vi "test_Split Registers by Direction_Errors.vi"(8 "error in (no error)":errorcluster, 11 "TestCase in":refnum<class "FPGA Addon Load And Parse Bitfile Unit Tests.lvclass">) -> (0 "error out":errorcluster, 3 "TestCase out":refnum<class "FPGA Addon Load And Parse Bitfile Unit Tests.lvclass">)   [LabVIEW 2018, in "FPGA Addon Load And Parse Bitfile Unit Tests.lvclass"]
uses:
  FPGA Addon Load And Parse Bitfile Unit Tests.lvclass
  <vilib>/addons/_JKI Toolkits/VI Tester/TestCase.llb/TestCase.lvclass
  Addon/Addon System Explorer/FPGA Addon System Explorer.lvlib
  C:/Program Files (x86)/National Instruments/LabVIEW 2018/vi.lib/addons/_JKI Toolkits/VI Tester/TestCase.llb/TestCase.lvclass
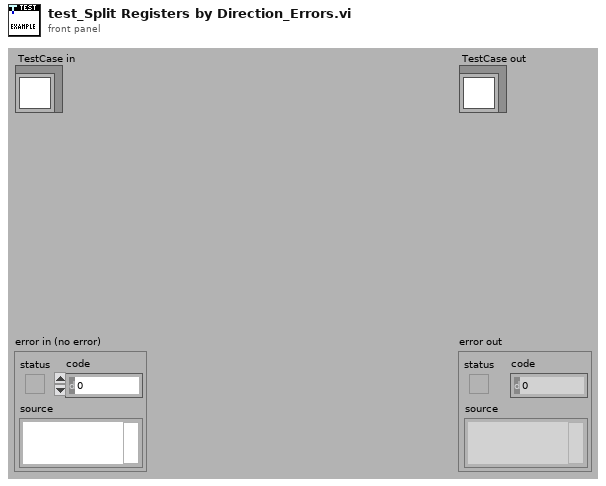
[diagram p1: front panel]
types:
  T1 = typedef "niFpgaBitfileStructure_VI.ctl" = cluster{"Name":string, "RegisterMap":T2[], "Icon":T7}
  T2 = typedef "nirviControlStructure.ctl" = cluster{"Name":string, "Hidden":bool, "Indicator":bool, "Flattened Type":string, "Grouping":cluster{"Grouped":bool, "Member Names":string[], "Member IDs":u32[]}, "Address":u32, "Size":u32, "Class":u32, "Internal":bool, "Typedef":T3, "ID":u32, "Bidirectional":bool, "Synchronous":bool, "Mechanical Action":T4, "Sub Controls":T5[], "Access May Timeout":bool, "Register Node":bool}
  T3 = typedef "nirviTypdefDescription.ctl" = cluster{"Typedef":bool, "Path":path}
  T4 = typedef "nirviMechanicalAction.ctl" = enum8{"Switch When Pressed", "Switch When Released", "Switch Until Released", "Latch When Pressed", "Latch When Released", "Latch Until Released"}
  T5 = typedef "nirviSubControlStructure.ctl" = cluster{"Name":string, "flattened Type":string, "Cluster Information":T6, "Typedef":T3}
  T6 = typedef "nirviClusterElementControl.ctl" = cluster{"Name Hierarchy":string[], "Item Order":u32[]}
  T7 = typedef "imagedata.ctl" = cluster{"image type":i32, "image depth":i32, "image":u8[], "mask":u8[], "colors":u32[], "Rectangle":cluster{"left":i16, "top":i16, "right":i16, "bottom":i16}}
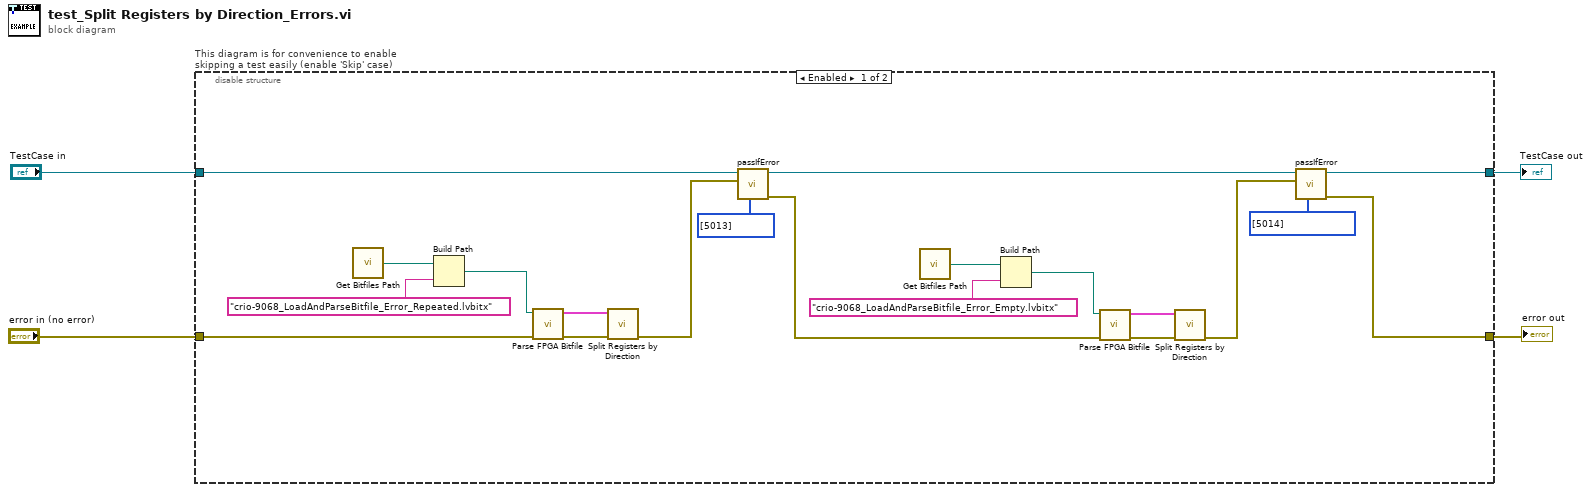
[diagram p0: block diagram]
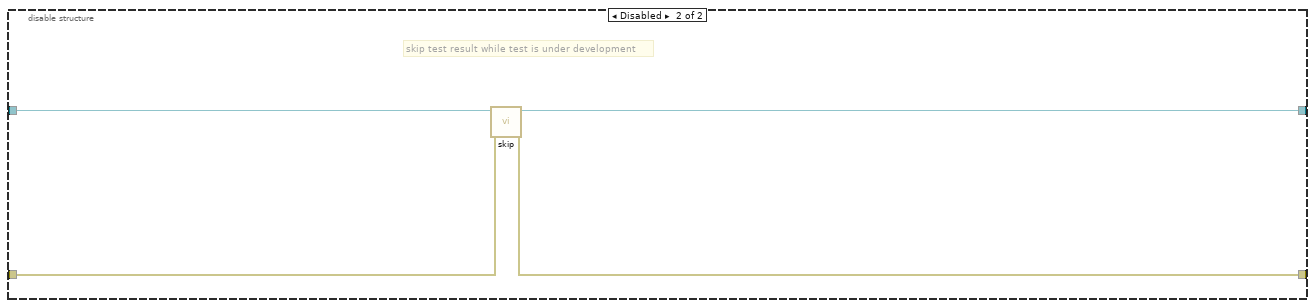
[diagram p2: hidden frame]
diagram:
  n1 = disable-structure "This diagram is for convenience to enable skipping a test easily (enable 'Skip' case)" shown="Enabled" {
    disable-tunnel: "TestCase in" -> [w18 w28]
    disable-tunnel: [w5 w26] -> w1
    disable-tunnel: [w6 w27] -> w3
    disable-tunnel: "error in (no error)" -> [w24 w25]
    frame Enabled {
      n2 = call "Get Bitfiles Path.vi"() -> ("Bitfiles path"=w21:path)
      n3 = Build Path(base path=w21, name or relative path="crio-9068_LoadAndParseBitfile_Error_Repeated.lvbitx") -> (appended path=w19:path)
      n4 = call "Parse FPGA Bitfile.vi"("error in (no error)"=w24, "Path"=w19) -> ("error out"=w23:errorcluster, "vi info"=w22:T1)  [unwired: 7 in, 1 out]
      n5 = call "Split Registers by Direction.vi"("error in"=w23, "vi info"=w22) -> ("error out"=w17:errorcluster)  [unwired: 7 in, 2 out]
      n6 = call-dynamic "passIfError.vi"("passing error codes (default = any error code)"=i32[] [5013], "error"=w17, "TestCase in"=w18) -> ("error out"=w10:errorcluster, "TestCase out"=w9:refnum<class "FPGA Addon Load And Parse Bitfile Unit Tests.lvclass">)  [unwired: 7 in]
      n7 = call "Get Bitfiles Path.vi"() -> ("Bitfiles path"=w13:path)
      n8 = Build Path(base path=w13, name or relative path="crio-9068_LoadAndParseBitfile_Error_Empty.lvbitx") -> (appended path=w11:path)
      n9 = call "Parse FPGA Bitfile.vi"("error in (no error)"=w10, "Path"=w11) -> ("error out"=w15:errorcluster, "vi info"=w14:T1)  [unwired: 7 in, 1 out]
      n10 = call "Split Registers by Direction.vi"("error in"=w15, "vi info"=w14) -> ("error out"=w8:errorcluster)  [unwired: 7 in, 2 out]
      n11 = call-dynamic "passIfError.vi"("passing error codes (default = any error code)"=i32[] [5014], "error"=w8, "TestCase in"=w9) -> ("error out"=w6:errorcluster, "TestCase out"=w5:refnum<class "FPGA Addon Load And Parse Bitfile Unit Tests.lvclass">)  [unwired: 7 in]
    }
    frame Disabled {
      # "skip test result while test is under development"
      n12 = call <vilib>:"skip.vi"("error in (no error)"=w25, "TestCase in"=w28) -> ("error out"=w27:errorcluster, "TestCase out"=w26:refnum<class "FPGA Addon Load And Parse Bitfile Unit Tests.lvclass">)  [unwired: 8 in]
    }
  }
  "error out" <- w3
  "TestCase out" <- w1
